vi "uxdesign.vi"() -> ()   [LabVIEW 2020]
panel:
  in  "stop":bool
  out "return value":string
  out "error out":errorcluster
  out "millisecond timer value":u32
  out "Action":string
  in  "Enum":enum16{"Device A", "Device B", "UBD5"}(ring)
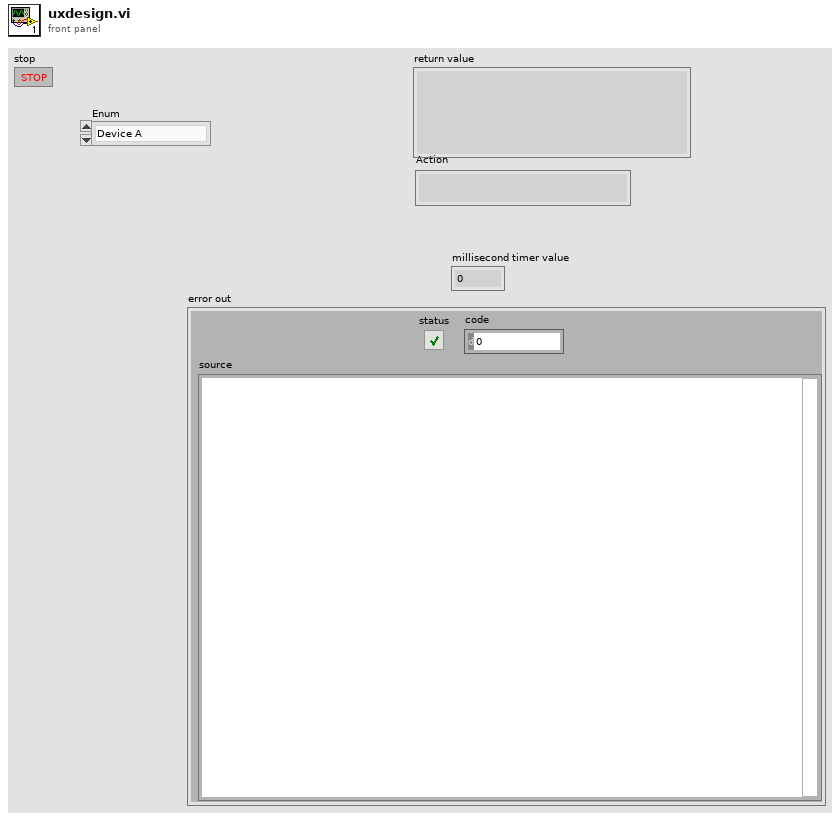
[diagram p1: front panel]
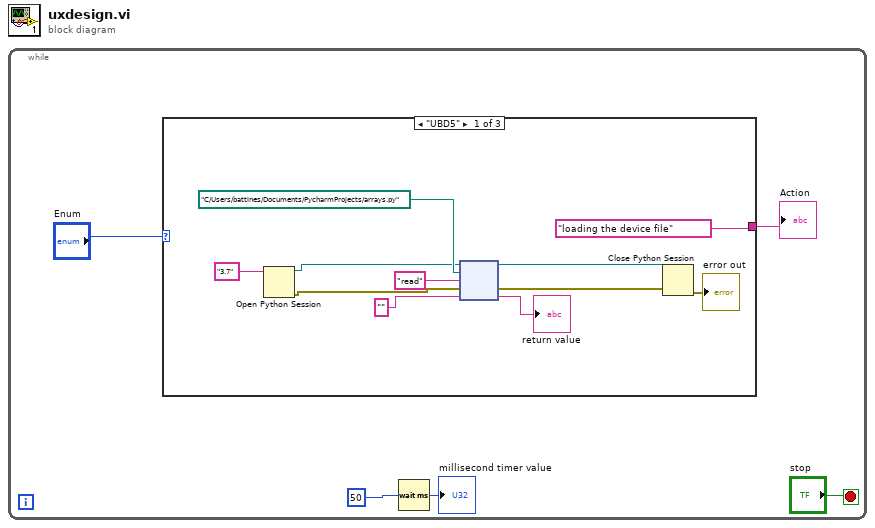
[diagram p0: block diagram]
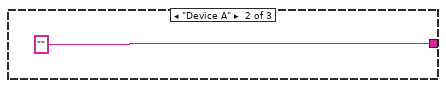
[diagram p2: hidden frame]
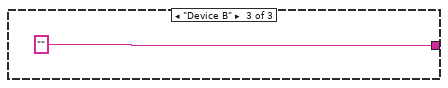
[diagram p3: hidden frame]
diagram:
  n1 = while {
    stop <- "stop" stop-if-true
    n2 = case shown="\"UBD5\"" "Enum" {
      tunnel: ["loading the device file" "" ""] -> w5
      frame "UBD5" {
        n3 = Open Python Session(python version="3.7" ("Python version")) -> (session out=w6:refnum<k35>, error out=w7:errorcluster)  [unwired: 2 in]
        n4 = node(w6, path "C:/Users/battines/Documents/PycharmProjects/arrays.py" ("module path"), "read" ("function name"), w7, "") -> (w15:refnum<k35>, w16:errorcluster, →"return value":string)  [unwired: 2 out]
        n5 = Close Python Session(session in=w15, error in=w16) -> (11:→"error out":errorcluster)
      }
      frame "Device A" {
      }
      frame "Device B" {
      }
    }
    "Action" <- w5
    n6 = Wait (ms)(milliseconds to wait=u32 50) -> (millisecond timer value=→"millisecond timer value":u32)
  }
